vi "AssemblyState.vi"(0 "error in":errorcluster, 3 "node":string) -> (1 "error out":errorcluster, 4 "Assembly State":T1)   [LabVIEW 2012]
uses:
  ROS/Code/SubVIs/_ROSDirection.ctl
  ROS/Code/Console/Servers/ServerSubs/TopicDef.ctl
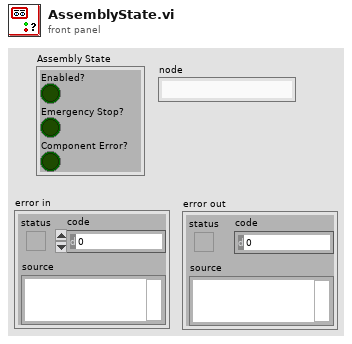
[diagram p1: front panel]
types:
  T1 = cluster{"Enabled?":bool, "Emergency Stop?":bool, "Component Error?":bool}
  T2 = typedef "TopicDef.ctl" = cluster{"Topic":string, "Type":string, "Action":T3, "Update (ms)":u16, "queue size":u16}
  T3 = typedef "_ROSDirection.ctl" = enum16{"Node", "Publisher", "Subscriber", "ServiceClient", "ServiceProvider"}
  T4 = typedef "_ROSControl.ctl" = cluster{"topic port":u16, "Node":string, "topic":string, "type":string, "node port":u16, "error ":errorcluster, "Direction":T3, "Update (ms)":u16, "FIFO size":u16}
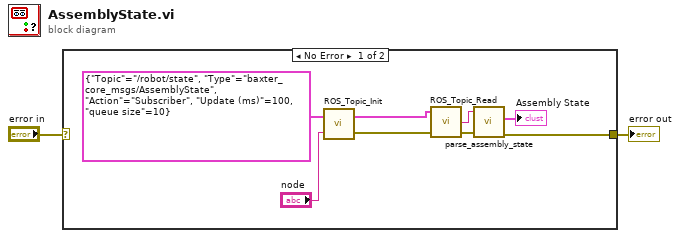
[diagram p0: block diagram]
diagram:
  n1 = case shown="No Error" "error in" {
    selector: "error in" -> [_ w11]
    tunnel: [w3 w11] -> w2
    frame No Error {
      n2 = call "ROS_Topic_Init.vi"("node"="node", "Definitions"=T2 {"Topic"="/robot/state", "Type"="baxter_core_msgs/AssemblyState", "Action"=enum."Subscriber", "Update (ms)"=100, "queue size"=10}) -> ("error out"=w5:errorcluster, "ROS out"=w8:T4)
      n3 = call "ROS_Topic_Read.vi"("error in (no error)"=w5, "ROS in"=w8) -> ("error out"=w4:errorcluster, "Reply"=w7:string)  [unwired: 1 in, 1 out]
      n4 = call "parse_assembly_state.vi"("Msg in"=w7, "error in"=w4) -> ("Assembly State"=→"Assembly State":T1, "error out"=w3:errorcluster)  [unwired: 1 in, 2 out]
    }
    frame Error {
    }
  }
  "error out" <- w2
